vi "2022_Version.vi"() -> ()   [LabVIEW 2022 SP3]
uses:
  <vilib>/ErrorRing/Error Ring.xnode
panel:
  in  "Instructions":bool
  out "Test":string
  out "Index_Display":i32
  out "Score":i32
  in  "Start Button":bool
  in  "Boolean 4":bool
  in  "Boolean 3":bool
  in  "Boolean 2":bool
  in  "Boolean":bool
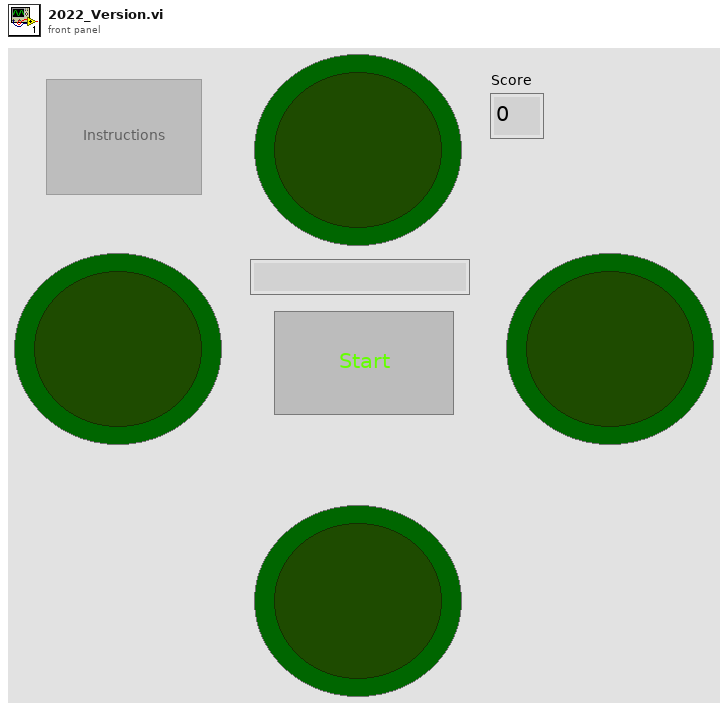
[diagram p1: front panel]
types:
  T1 = enum16{"Default", "Initialization", "New Random", "Display", "Player Choice", "IsCorrect", "Loss", "Error_Case", "Instructions"}
  T2 = enum8{"Enabled", "Disabled", "Disabled and Grayed Out"}
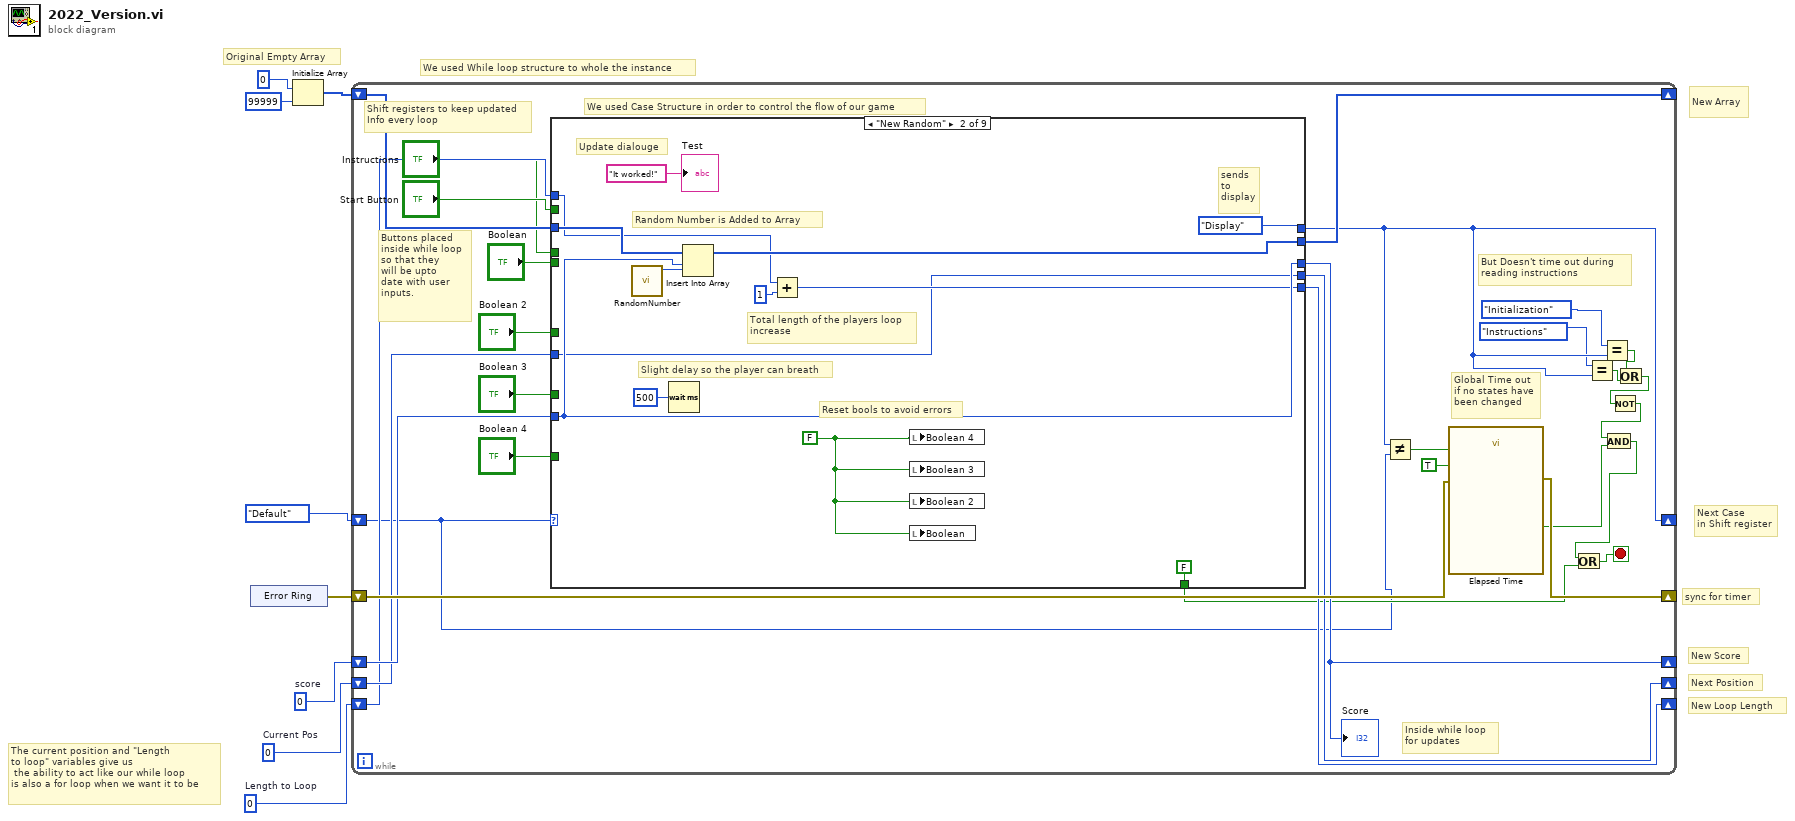
[diagram p0: block diagram]
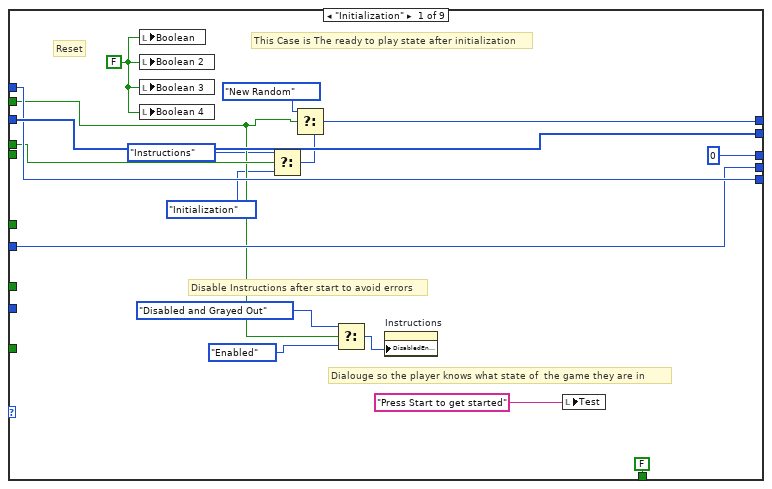
[diagram p2: hidden frame]
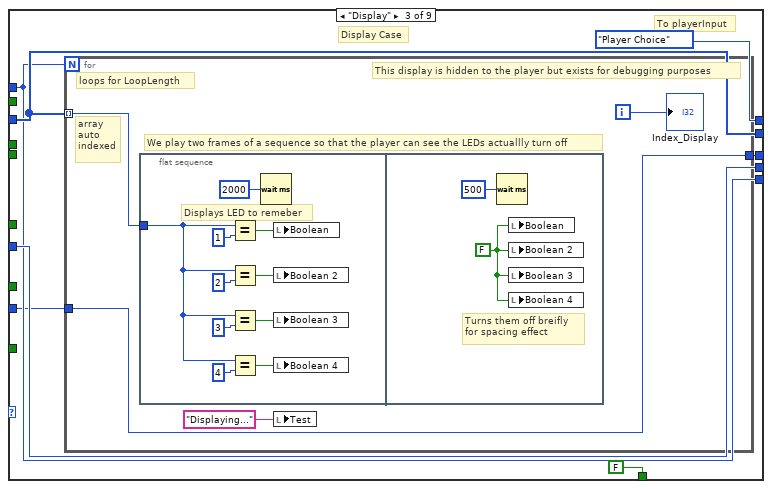
[diagram p3: hidden frame]
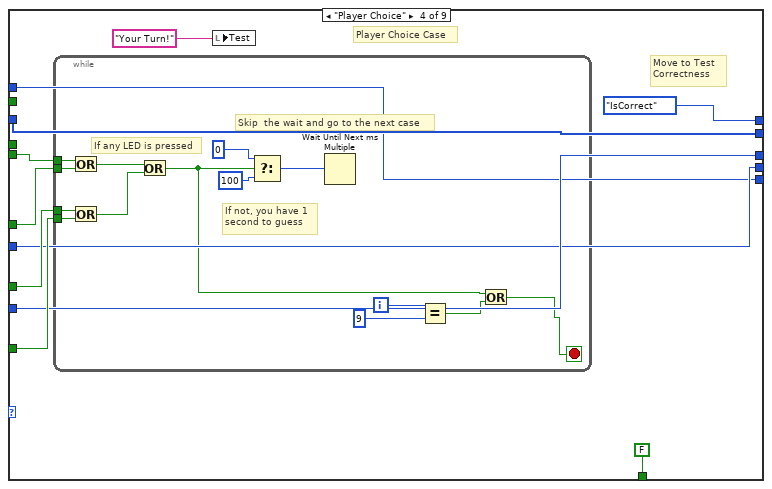
[diagram p4: hidden frame]
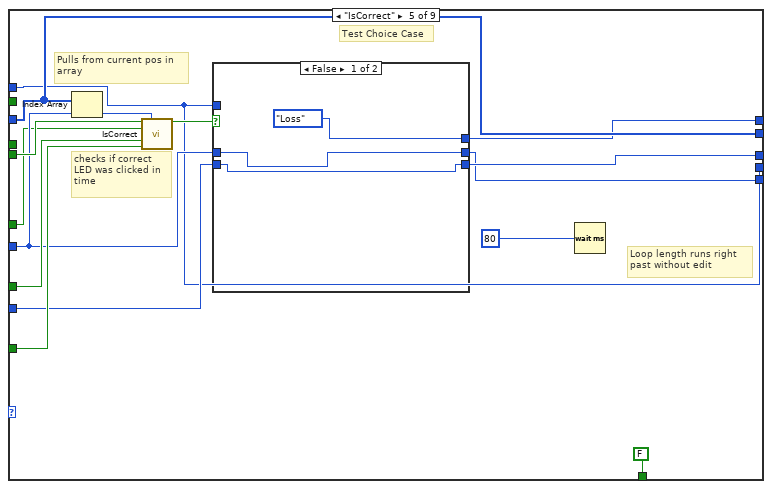
[diagram p5: hidden frame]
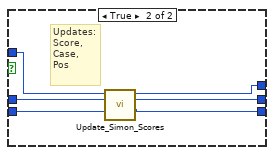
[diagram p6: hidden frame]
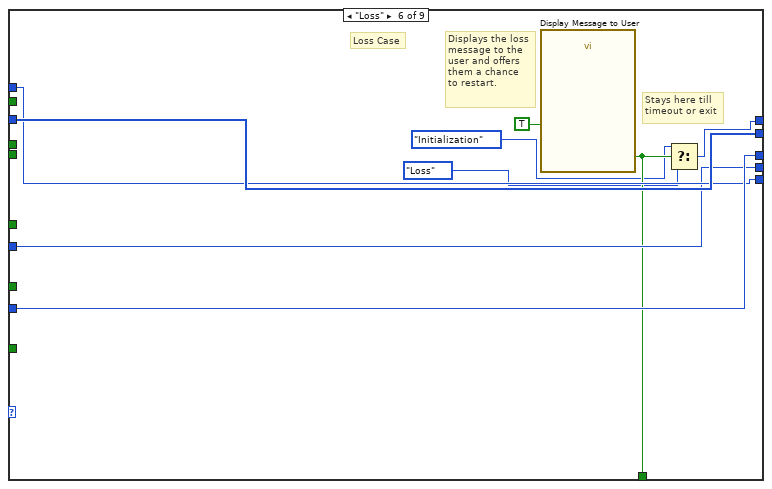
[diagram p7: hidden frame]
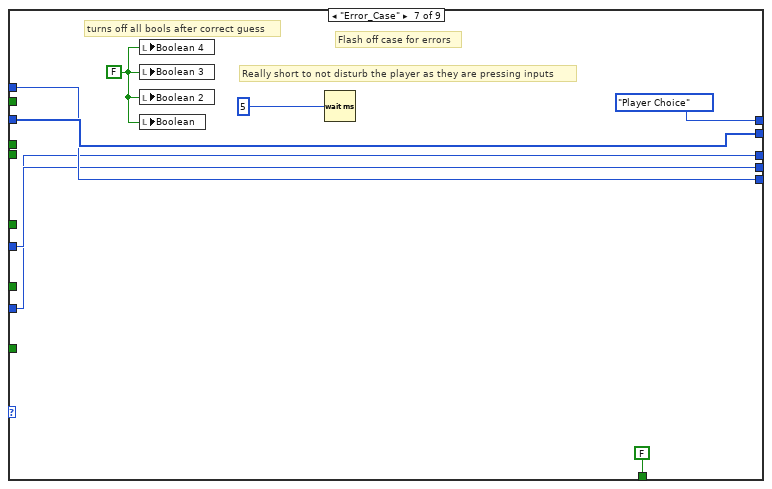
[diagram p8: hidden frame]
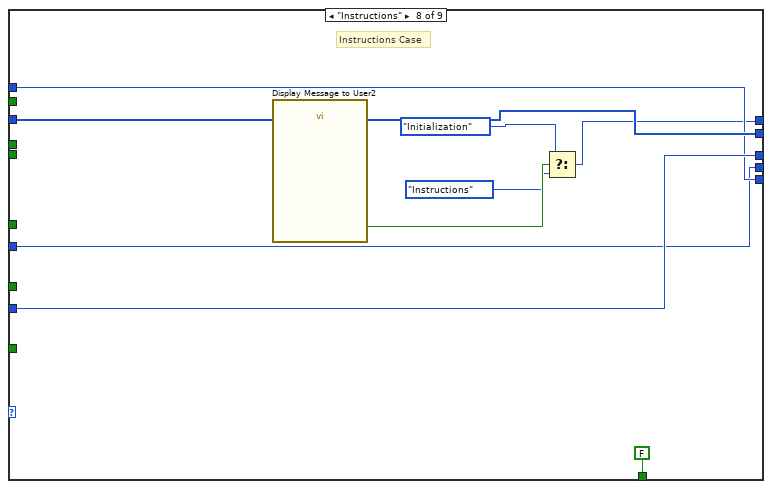
[diagram p9: hidden frame]
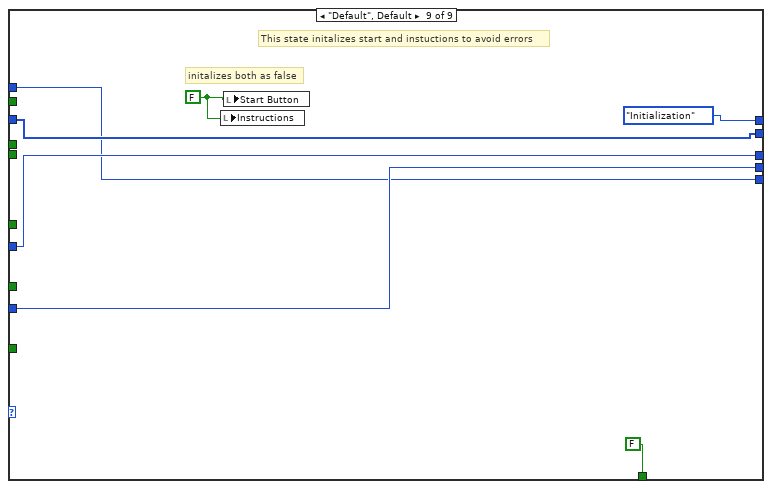
[diagram p10: hidden frame]
diagram:
  w3 = 0  # Length to Loop
  w4 = 0  # Current Pos
  w8 = 0  # score
  # "We used While loop structure to whole the instance"
  # "sync for timer"
  # "New Loop Length"
  # "Next Position"
  # "New Score"
  # "Next Case\nin Shift register"
  # "New Array"
  # "The current position and \"Length \nto loop\" variables give us\n the ability to act like our while loop\nis also a for loop when we want it to be"
  # "Original Empty Array"
  n1 = xnode "Error Ring"() -> ("error out"=w2:errorcluster)
  n2 = Initialize Array(0 ("element"), 99999 ("dimension size")) -> (w5:i32[])
  n3 = while {
    shift-right: [w36] -> _
    shift-left: w2 -> [w35]
    shift-right: [w31] -> _
    shift-left: w8 -> [w33]
    shift-right: [w32] -> _
    shift-left: w5 -> [w34]
    shift-right: [w28] -> _
    shift-left: w3 -> [w29]
    shift-right: [w27] -> _
    shift-left: w4 -> [w30]
    shift-right: [w11] -> _
    shift-left: T1."Default" -> [w12]
    stop <- w14 stop-if-true
    # "We used Case Structure in order to control the flow of our game"
    # "But Doesn't time out during\nreading instructions"
    # "Global Time out\nif no states have\nbeen changed"
    # "Inside while loop \nfor updates"
    # "Buttons placed\ninside while loop\nso that they \nwill be upto\ndate with user\ninputs."
    # "Shift registers to keep updated \nInfo every loop"
    n4 = case shown="\"New Random\"" w12 {
      tunnel: "Start Button" -> [w47 _ _ _ _ _ _ _ _]
      tunnel: w34 -> [w54 w68 w75 w98 w124 w149 w157 w164 w173]
      tunnel: w33 -> [_ w64 w71 w97 w127 w147 w154 w165 w171]
      tunnel: [w54 w67 w75 w98 w124 w149 w157 w164 w173] -> w32
      tunnel: [0 ("score") w64 w72 w97 w126 w147 w154 w165 w172] -> w31
      tunnel: "Boolean" -> [_ _ _ w102 w131 _ _ _ _]
      tunnel: "Boolean 2" -> [_ _ _ w101 w119 _ _ _ _]
      tunnel: "Boolean 3" -> [_ _ _ w100 w130 _ _ _ _]
      tunnel: "Boolean 4" -> [_ _ _ w99 w129 _ _ _ _]
      tunnel: w30 -> [w52 w60 w74 w96 w123 w145 w155 w162 w172]
      tunnel: w29 -> [w53 w63 w73 w95 w121 w146 w156 w163 w170]
      tunnel: [w53 w61 w73 w95 w121 w146 w156 w163 w170] -> w28
      tunnel: [w52 w60 w74 w96 w122 w145 w155 w162 w171] -> w27
      tunnel: "Instructions" -> [w49 _ _ _ _ _ _ _ _]
      tunnel: [FALSE ("OK") FALSE ("OK") FALSE ("OK") FALSE ("OK") FALSE ("OK") w144 FALSE ("OK") FALSE ("OK") FALSE ("OK")] -> w15
      tunnel: [w39 T1."Display" T1."Player Choice" T1."IsCorrect" w117 w141 T1."Player Choice" w158 T1."Initialization"] -> w11
      frame "Initialization" {
        w51 = FALSE ("Boolean")
        # "Disable Instructions after start to avoid errors"
        # "Dialouge so the player knows what state of  the game they are in"
        # "This Case is The ready to play state after initialization"
        # "Reset"
        n5 = local write "Boolean"(w51) -> ()
        n6 = local write "Boolean 2"(w51) -> ()
        n7 = local write "Boolean 3"(w51) -> ()
        n8 = local write "Boolean 4"(w51) -> ()
        n9 = Select(t=T1."Instructions", s=w49, f=T1."Initialization") -> (s? t:f=w48:T1)
        n10 = Select(t=T1."New Random", s=w47, f=w48) -> (s? t:f=w39:T1)
        n11 = Select(t=T2."Disabled and Grayed Out" ("Disabled"), s=w47, f=T2."Enabled" ("Disabled")) -> (s? t:f=w44:T2)
        n12 = property on="Instructions" class="Bool (strict)"("DisabledEnum"=w44) -> ()  [unwired: 2 in, 2 out]
        n13 = local write "Test"("Press Start to get started" ("Test")) -> ()
      }
      frame "New Random" {
        w58 = FALSE ("Boolean 4")
        # "sends\nto\ndisplay"
        # "Reset bools to avoid errors"
        # "Slight delay so the player can breath"
        # "Total length of the players loop\nincrease"
        # "Random Number is Added to Array"
        # "Update dialouge"
        n14 = call "RandomNumber.vi"() -> ("Numeric"=w66:i32)  [unwired: 11 in]
        n15 = Wait (ms)(milliseconds to wait=u32 500) -> ()  [unwired: 1 out]
        n16 = Insert Into Array(array=w68, index=w64, new element=w66) -> (w67:i32[])
        n17 = Add(x=w63, y=1) -> (x+y=w61:i32)
        n18 = local write "Boolean 4"(w58) -> ()
        n19 = local write "Boolean 3"(w58) -> ()
        n20 = local write "Boolean 2"(w58) -> ()
        n21 = local write "Boolean"(w58) -> ()
        "Test" <- "It worked!"
      }
      frame "Display" {
        # "Display Case"
        # "To playerInput"
        n22 = for {
          N: w73 -> [_]
          tunnel: w75 -> [w78] mode=indexing
          tunnel: w71 -> [w77]
          tunnel: [w77] -> w72
          i -> [w79]
          # "array\nauto\nindexed"
          # "loops for LoopLength"
          # "We play two frames of a sequence so that the player can see the LEDs actuallly turn off"
          # "This display is hidden to the player but exists for debugging purposes"
          n23 = flat-sequence {
            tunnel: w78 -> [w83]
            frame #0 {
              # "Displays LED to remeber"
              n24 = Equal?(x=w83, y=1) -> (x = y?=w89:bool)
              n25 = Equal?(x=w83, y=2) -> (x = y?=w86:bool)
              n26 = Equal?(x=w83, y=3) -> (x = y?=w87:bool)
              n27 = Equal?(x=w83, y=4) -> (x = y?=w88:bool)
              n28 = Wait (ms)(milliseconds to wait=u32 2000) -> ()  [unwired: 1 out]
              n29 = local write "Boolean"(w89) -> ()
              n30 = local write "Boolean 2"(w86) -> ()
              n31 = local write "Boolean 3"(w87) -> ()
              n32 = local write "Boolean 4"(w88) -> ()
            }
            frame #1 {
              w91 = FALSE ("Boolean 4")
              # "Turns them off breifly \nfor spacing effect"
              n33 = Wait (ms)(milliseconds to wait=u32 500 ("x")) -> ()  [unwired: 1 out]
              n34 = local write "Boolean"(w91) -> ()
              n35 = local write "Boolean 2"(w91) -> ()
              n36 = local write "Boolean 3"(w91) -> ()
              n37 = local write "Boolean 4"(w91) -> ()
            }
          }
          n38 = local write "Test"("Displaying..." ("Test")) -> ()
          "Index_Display" <- w79
        }
      }
      frame "Player Choice" {
        # "Move to Test \nCorrectness"
        # "Player Choice Case"
        n39 = while {
          tunnel: w102 -> [w114]
          tunnel: w101 -> [w113]
          tunnel: w100 -> [w112]
          tunnel: w99 -> [w111]
          i -> [w107]
          stop <- w105 stop-if-true
          # "If not, you have 1\nsecond to guess"
          # "Skip  the wait and go to the next case"
          # "If any LED is pressed"
          n40 = Or(x=w114, y=w113) -> (x .or. y?=w116:bool)
          n41 = Or(x=w112, y=w111) -> (x .or. y?=w115:bool)
          n42 = Or(x=w116, y=w115) -> (x .or. y?=w103:bool)
          n43 = Select(t=u32 0 ("milliseconds to wait"), s=w103, f=u32 100 ("milliseconds to wait")) -> (s? t:f=w108:u32)
          n44 = Wait Until Next ms Multiple(millisecond multiple=w108) -> ()  [unwired: 1 out]
          n45 = Equal?(x=w107, y=9) -> (x = y?=w104:bool)
          n46 = Or(x=w103, y=w104) -> (x .or. y?=w105:bool)
        }
        n47 = local write "Test"("Your Turn!" ("Test")) -> ()
      }
      frame "IsCorrect" {
        # "Test Choice Case"
        # "Pulls from current pos in\narray"
        # "Loop length runs right \npast without edit"
        # "checks if correct\nLED was clicked in\ntime"
        n48 = Index Array(array=w124, index=w123) -> (element=w128:i32)
        n49 = call "IsCorrect.vi"("Boolean"=w131, "InValue"=w128, "Boolean 2"=w119, "Boolean 3"=w130, "Boolean 4"=w129) -> ("IsCorrect"=w125:bool)  [unwired: 10 in]
        n50 = case shown="False" w125 {
          tunnel: w127 -> [w134 w138]
          tunnel: [w134 w137] -> w126
          tunnel: w123 -> [w133 w139]
          tunnel: [w133 w136] -> w122
          tunnel: w121 -> [_ w140]
          tunnel: [T1."Loss" w135] -> w117
          frame False {
          }
          frame True {
            # "Updates:\nScore,\nCase,\nPos"
            n51 = call "Update_Simon_Scores.vi"("Score"=w138, "Position"=w139, "LoopLength"=w140) -> ("New Score"=w137:i32, "Next Pos"=w136:i32, "Case Selector out"=w135:T1)  [unwired: 6 in]
          }
        }
        n52 = Wait (ms)(milliseconds to wait=u32 80) -> ()  [unwired: 1 out]
      }
      frame "Loss" {
        # "Loss Case"
        # "Stays here till\ntimeout or exit"
        # "Displays the loss\nmessage to the \nuser and offers\nthem a chance \nto restart."
        n53 = call "Display Message to User"("Enable"=TRUE) -> ("OK"=w144:bool)  [unwired: 9 in, 1 out]
        n54 = Select(t=T1."Initialization", s=w144, f=T1."Loss") -> (s? t:f=w141:T1)
      }
      frame "Error_Case" {
        w153 = FALSE ("Boolean 4")
        # "turns off all bools after correct guess"
        # "Really short to not disturb the player as they are pressing inputs"
        # "Flash off case for errors"
        n55 = local write "Boolean 4"(w153) -> ()
        n56 = local write "Boolean 3"(w153) -> ()
        n57 = local write "Boolean 2"(w153) -> ()
        n58 = local write "Boolean"(w153) -> ()
        n59 = Wait (ms)(milliseconds to wait=u32 5) -> ()  [unwired: 1 out]
      }
      frame "Instructions" {
        # "Instructions Case"
        n60 = call "Display Message to User2"() -> ("OK"=w166:bool)  [unwired: 10 in, 1 out]
        n61 = Select(t=T1."Initialization", s=w166, f=T1."Instructions") -> (s? t:f=w158:T1)
      }
      frame "Default", Default {
        w169 = FALSE ("Start Button")
        # "initalizes both as false"
        # "This state initalizes start and instuctions to avoid errors"
        n62 = local write "Instructions"(w169) -> ()
        n63 = local write "Start Button"(w169) -> ()
      }
    }
    "Score" <- w31
    n64 = Not Equal?(x=w11, y=w12) -> (x != y?=w37:bool)
    n65 = call "Elapsed Time"("Reset"=w37, "Auto Reset"=TRUE, "error in (no error)"=w35) -> ("Time has Elapsed"=w20:bool, "error out"=w36:errorcluster)  [unwired: 9 in, 6 out]
    n66 = Equal?(x=T1."Instructions", y=w11) -> (x = y?=w19:bool)
    n67 = Equal?(x=T1."Initialization", y=w11) -> (x = y?=w18:bool)
    n68 = Or(x=w18, y=w19) -> (x .or. y?=w17:bool)
    n69 = Not(x=w17) -> (.not. x?=w16:bool)
    n70 = And(x=w16, y=w20) -> (x .and. y?=w13:bool)
    n71 = Or(x=w13, y=w15) -> (x .or. y?=w14:bool)
  }
